vi "ESN_OfflineTraining.vi"(8 "error in (no error)":errorcluster, 9 "I/O pairs":cluster{"Input":dbl[], "Output":dbl[]}[](array[cluster]), 11 "ESN Status":T1) -> (0 "error out":errorcluster, 3 "ESN trained":T1)   [LabVIEW 2017]
uses:
  ESN_Network.ctl
  <vilib>/Analysis/Matrix/Datatypes/RealMatrix.ctl
  <vilib>/Analysis/_algsub.llb/Real PseudoInverse Matrix.vi
  <vilib>/Analysis/baseanly.llb/Real A x B.vi
  <vilib>/Analysis/7linalg.llb/Real Transpose Matrix.vi
  <vilib>/Analysis/Matrix/Numeric/Conversions/Array To Matrix - RA2.vi
  <vilib>/Analysis/NI_AALPro.lvlib
  <vilib>/Analysis/NI_AALBase.lvlib
  <vilib>/Analysis/Matrix/NI_Matrix.lvlib
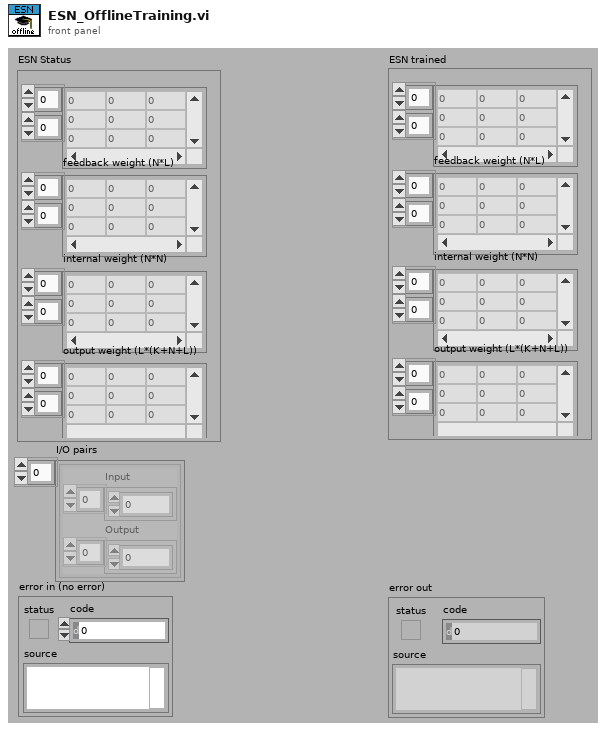
[diagram p1: front panel]
types:
  T1 = typedef "ESN_Network.ctl" = cluster{"output to internal feedback?":bool, "output to output feedback?":bool, "input to output feedforward?":bool, "number of input (K)":i32, "number of internal (N)":i32, "number of output (L)":i32, "input normalization vector":dbl[], "output restore vector":dbl[], "input weight (N*K)":T2, "feedback weight (N*L)":T2, "internal weight (N*N)":T2, "output weight (L*(K+N+L))":T2}
  T2 = typedef "NI_Matrix.lvlib/RealMatrix.ctl" = dbl[][]
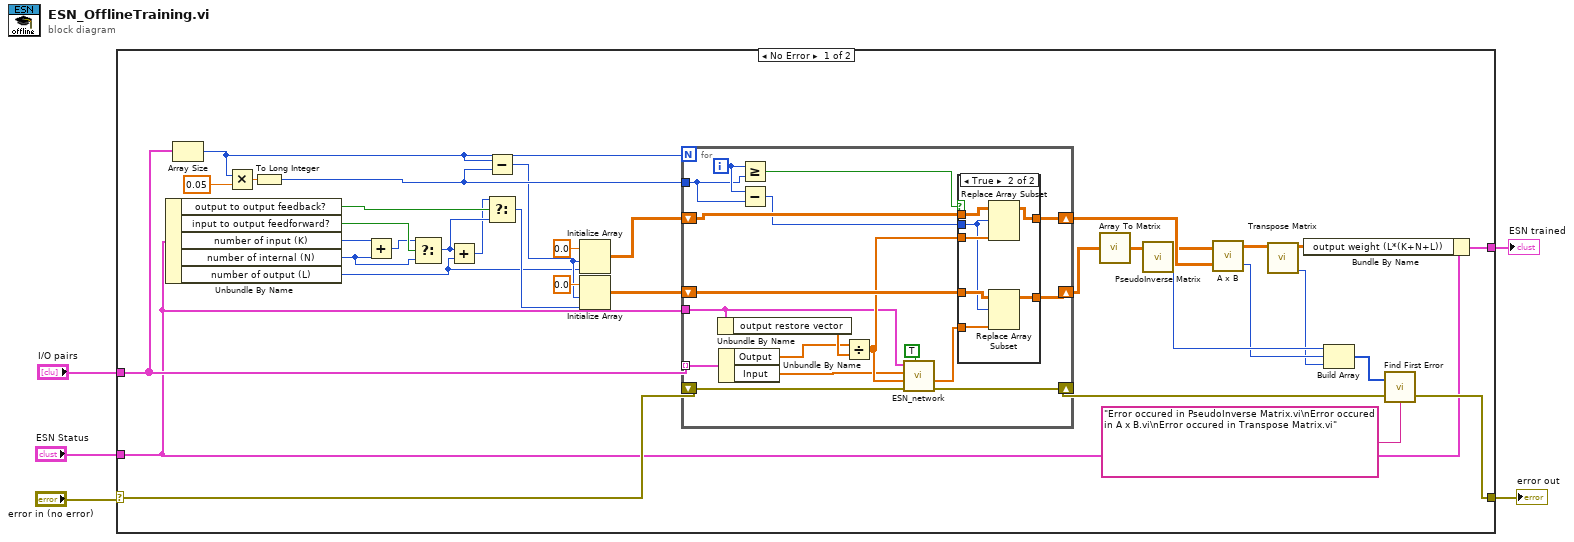
[diagram p0: block diagram]
diagram:
  n1 = case shown="No Error" "error in (no error)" {
    selector: "error in (no error)" -> [w34 w68]
    tunnel: "I/O pairs" -> [w40 _]
    tunnel: "ESN Status" -> [w26 _]
    tunnel: [w35 _] -> w3
    tunnel: [w27 w68] -> w1
    frame No Error {
      n2 = Unbundle By Name(w26) -> ("output to output feedback?"=w24:bool, "input to output feedforward?"=w23:bool, "number of input (K)"=w25:i32, "number of internal (N)"=w22:i32, "number of output (L)"=w11:i32)
      n3 = Array Size(array=w40) -> (size(s)=w18:i32)
      n4 = Multiply(x=w18, y=0.05) -> (x*y=w38:dbl)
      n5 = To Long Integer(number=w38) -> (32bit integer=w17:i32)
      n6 = Add(x=w25, y=w22) -> (x+y=w21:i32)
      n7 = Select(t=w21, s=w23, f=w22) -> (s? t:f=w20:i32)
      n8 = Add(x=w20, y=w11) -> (x+y=w19:i32)
      n9 = Subtract(x=w18, y=w17) -> (x-y=w12:i32)
      n10 = Select(t=w19, s=w24, f=w20) -> (s? t:f=w15:i32)
      n11 = Initialize Array(0.0 ("element"), w12, w11) -> (w10:dbl[][])
      n12 = Initialize Array(0.0 ("element"), w12, w15) -> (w14:dbl[][])
      n13 = for {
        N: w18 -> [_]
        tunnel: w40 -> [w58] mode=indexing
        tunnel: w26 -> [w44]
        shift-right: [w57] -> w9
        shift-left: w10 -> [w56]
        tunnel: w17 -> [w42]
        shift-right: [w54] -> w7
        shift-left: w14 -> [w53]
        shift-right: [w50] -> w29
        shift-left: w34 -> [w51]
        i -> [w43]
        n14 = Unbundle By Name(w44) -> ("output restore vector"=w49:dbl[])
        n15 = Unbundle By Name(w58) -> ("Output"=w47:dbl[], "Input"=w45:dbl[])
        n16 = Greater Or Equal?(x=w43, y=w42) -> (x >= y?=w55:bool)
        n17 = Subtract(x=w43, y=w42) -> (x-y=w41:i32)
        n18 = Divide(x=w47, y=w49) -> (x/y=w46:dbl[])
        n19 = call "ESN_network.vi"("In train phase? (F)"=TRUE ("In train phase?"), "error in (no error)"=w51, "Desired output"=w46, "input"=w45, "ESN Status"=w44) -> ("error out"=w50:errorcluster, "State collection"=w48:dbl[])  [unwired: 3 in, 2 out]
        n20 = case shown="True" w55 {
          tunnel: w46 -> [_ w63]
          tunnel: [w60 w66] -> w57
          tunnel: w56 -> [w60 w67]
          tunnel: w48 -> [_ w62]
          tunnel: [w59 w65] -> w54
          tunnel: w53 -> [w59 w64]
          tunnel: w41 -> [_ w61]
          frame False {
          }
          frame True {
            n21 = Replace Array Subset(array=w67, new element=w63, index (row)=w61) -> (w66:dbl[][])  [unwired: 1 in]
            n22 = Replace Array Subset(array=w64, new element=w62, index (row)=w61) -> (w65:dbl[][])  [unwired: 1 in]
          }
        }
      }
      n23 = call-poly <vilib>:"Array To Matrix.vi"("Real 2D Array"=w7) -> ("Real Matrix"=w6:T2)
      n24 = call-poly <vilib>:"PseudoInverse Matrix.vi"("Input Matrix"=w6) -> ("error"=w33:i32, "PseudoInverse Matrix"=w8:T2)  [unwired: 1 in]
      n25 = call-poly <vilib>:"A x B.vi"("B"=w9, "A"=w8) -> ("error"=w32:i32, "A x B"=w37:T2)
      n26 = call-poly <vilib>:"Transpose Matrix.vi"("Input Matrix"=w37) -> ("error"=w31:i32, "Matrix Transpose"=w36:T2)  [unwired: 9 in]
      n27 = Bundle By Name(cluster=w26, "output weight (L*(K+N+L))"=w36) -> (w35:T1)
      n28 = Build Array(w33, w32, w31) -> (w30:i32[])
      n29 = call <vilib>:"Find First Error.vi"("error in (no error)"=w29, "source messages"="Error occured in PseudoInverse Matrix.vi\nError occured in A x B.vi\nError occured in Transpose Matrix.vi", "error codes"=w30) -> ("error out"=w27:errorcluster)  [unwired: 1 in, 1 out]
    }
    frame Error {
    }
  }
  "ESN trained" <- w3
  "error out" <- w1
